vi "48.vi"() -> ()   [LabVIEW 2021]
panel:
  out "Numeric":u64
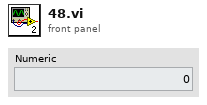
[diagram p1: front panel]
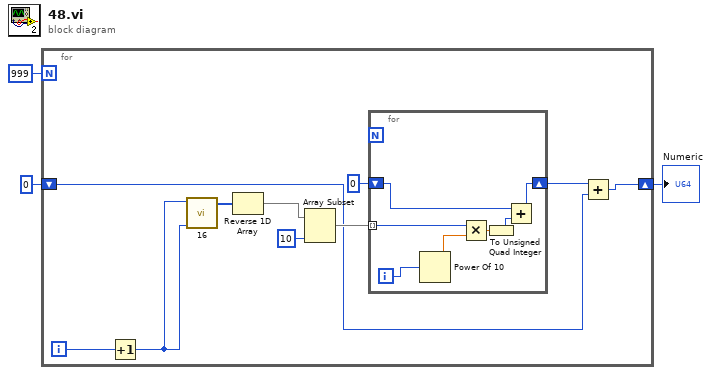
[diagram p0: block diagram]
diagram:
  n1 = for {
    N: 999 -> [_]
    shift-right: [w6] -> w2
    shift-left: u64 0 -> [w5]
    i -> [w13]
    n2 = Increment(x=w13) -> (x+1=w4:i32)
    n3 = call "16.vi"("base"=w4, "exponent"=w4) -> ("reversed array 2"=w12:u8[])  [unwired: 9 in]
    n4 = Reverse 1D Array(array=w12) -> (reversed array=w11:u8[])
    n5 = Array Subset(array=w11, length=10) -> (w9:u8[])  [unwired: 1 in]
    n6 = for {
      tunnel: w9 -> [w20] mode=indexing
      shift-right: [w14] -> w7
      shift-left: u64 0 -> [w15]
      i -> [w19]
      n7 = Power Of 10(x=w19) -> (10^x=w18:dbl)
      n8 = Multiply(x=w20, y=w18) -> (x*y=w17:dbl)
      n9 = To Unsigned Quad Integer(1:w17) -> (0:w16:u64)
      n10 = Add(x=w15, y=w16) -> (x+y=w14:u64)
    }
    n11 = Add(x=w7, y=w5) -> (x+y=w6:u64)
  }
  "Numeric" <- w2
